vi "Camera Manager Grab Char.vi"(8 "error in (no error)":errorcluster, 10 "imgPtr":string, 11 "cameraId":i32) -> (0 "error out":errorcluster, 2 "imgPtr out":string)   [LabVIEW 2017, in "PlayNitrideCameraComponet1010_4.lvlib"]
doc: "__declspec(dllexport) void CameraManager_Grab_Char(int cameraId, unsigned char* imgPtr);"
uses:
  <userlib>/PlayNitrideCameraComponet1010_4/PlayNitrideCameraComponet1010_4.lvlib
  <userlib>/PlayNitrideCameraComponet1010_4/PlayNitrideCameraComponet.dll
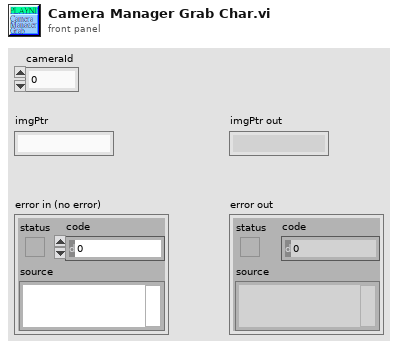
[diagram p1: front panel]
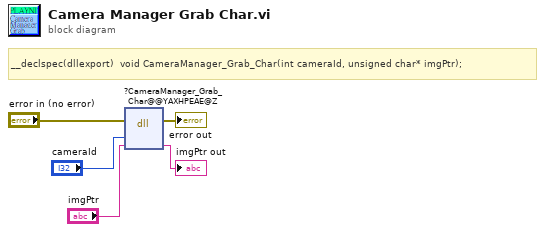
[diagram p0: block diagram]
diagram:
  # "__declspec(dllexport)  void CameraManager_Grab_Char(int cameraId, unsigned char* imgPtr);"
  n1 = dll-call lib="C:/Program Files/National Instruments/LabVIEW 2017/user.lib/PlayNitrideCameraComponet1010_4/PlayNitrideCameraComponet.*" fn="?CameraManager_Grab_Char@@YAXHPEAE@Z"(error in="error in (no error)", "cameraId"="cameraId", "imgPtr"="imgPtr") -> (error out=→"error out":errorcluster, "imgPtr"=→"imgPtr out":string)  [unwired: 4 in, 1 out]
